vi "hotch-YangZhang.vi"(0 "fs":dbl, 2 "f1":dbl, 3 "f2":dbl, 5 "R":dbl) -> (1 "reverse coefficients":dbl[](array[numeric]), 4 "forward coefficients":dbl[](array[numeric]), 6 "Magnitude":cluster{dbl[], dbl[]}(graph), 7 "Phase":cluster{dbl[], dbl[]}(graph), 8 "Pole-Zero Plot":cluster{dbl[], dbl[]}[](graph))   [LabVIEW 2016]
uses:
  <vilib>/imath/engines/lvmath2/RunTimeEngine/BuiltInFunctions/conv/NIMS_conv(V,V).vi
  <instcachedir>/0/NIMS_conv(V,V)_D3E194F2B5174935BB2368CEB7AAC5A9.lvgen/NIMS_conv(V,V)_D3E194F2B5174935BB2368CEB7AAC5A9_000.vi
  <vilib>/imath/engines/lvmath2/RunTimeEngine/ErrorHandling/NIMS_Error From Error Code.vi
  <vilib>/imath/engines/lvmath2/RunTimeEngine/NodeEndStatement/NIMS_NodeEndStatement_Output.vi
  <instcachedir>/0/NIMS_NodeEndStatement_Output_53EC0D466D134D7ABD903AC30B43404B.lvgen/NIMS_NodeEndStatement_Output_53EC0D466D134D7ABD903AC30B43404B_005.vi
  <vilib>/imath/engines/lvmath2/RunTimeEngine/ErrorHandling/NIMS_Finalize Error.vi
  Program Files (x86)/National Instruments/Scripts/Plot Pole-Zero - direct.vi
  Program Files (x86)/National Instruments/Scripts/Plot Frequency Response - direct.vi
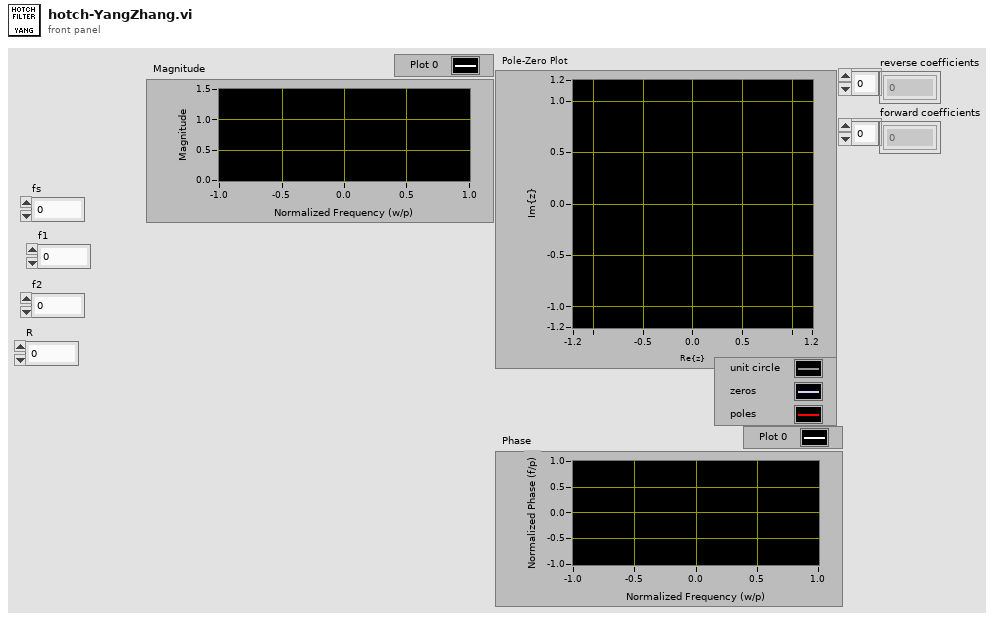
[diagram p1: front panel]
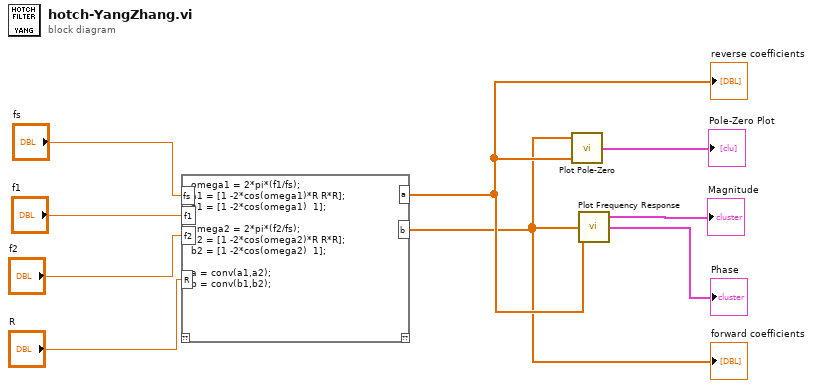
[diagram p0: block diagram]
diagram:
  n1 = mathscript code="omega1 = 2*pi*(f1/fs);\na1 = [1 -2*cos(omega1)*R R*R];\nb1 = [1 -2*cos(omega1)  1];\n\nomega2 = 2*pi*(f2/fs);\na2 = [1 -2*cos(omega2)*R R*R];\nb2 = [1 -2*cos(omega2)  1];\n\na = conv(a1,a2);\nb = conv(b1,b2);"("fs"="fs", "f1"="f1", "R"="R", "f2"="f2") -> ("a"=w5:dbl[], "b"=w4:dbl[])  [unwired: 1 in, 1 out]
  "reverse coefficients" <- w5
  "forward coefficients" <- w4
  n2 = call-poly "Plot Pole-Zero.vi"("a, reverse coefficients"=w5, "b, forward coefficients"=w4) -> ("Pole-Zero Plot"=→"Pole-Zero Plot":cluster{dbl[], dbl[]}[])  [unwired: 3 in]
  n3 = call-poly "Plot Frequency Response.vi"("b, forward coefficients"=w4, "a, reverse coefficients"=w5) -> ("Magnitude"=→"Magnitude":cluster{dbl[], dbl[]}, "Phase"=→"Phase":cluster{dbl[], dbl[]})  [unwired: 3 in, 1 out]
